vi "与副屏通信master.vi"() -> ()   [LabVIEW 2016, in "斯坦道多参数.lvlib"]
uses:
  <vilib>/NI/Modbus Library/API/Wrapper/Create TCP Master.vi
  <vilib>/NI/Modbus Library/API/master/Modbus Master.lvclass
  <vilib>/NI/Modbus Library/API/Wrapper/API Main.lvlib
  <vilib>/ptbypt/NI_PtbyPt.lvlib
panel:
  out "副屏启动命令":u16
  in  "停止 2":bool
  out "read values 2":u16[](array[numeric])
  in  "registers to write 2":u16[](array[numeric])
  out "error out 2":errorcluster caption="error out"
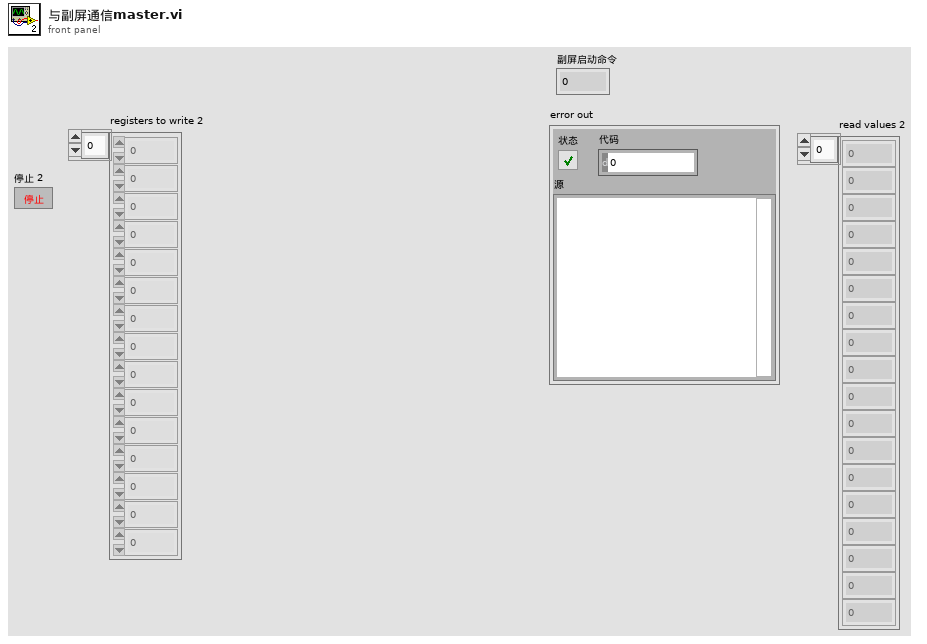
[diagram p1: front panel]
types:
  T1 = enum32{"Bad", "Idle", "Run top level", "Running"}
  T2 = cluster{"Boolean array[0]":bool, "Boolean array[1]":bool, "Boolean array[2]":bool, "Boolean array[3]":bool, "Boolean array[4]":bool, "Boolean array[5]":bool, "Boolean array[6]":bool, "Boolean array[7]":bool}
  T3 = cluster{"数据保存间隔":dbl, "保存组数":dbl, "水温标样值":dbl, "pH标样值":dbl, "溶解氧标样值":dbl, "电导率标样值":dbl, "浊度标样值":dbl, "pH启用":bool, "溶解氧启用":bool, "电导率启用":bool, "浊度启用":bool}
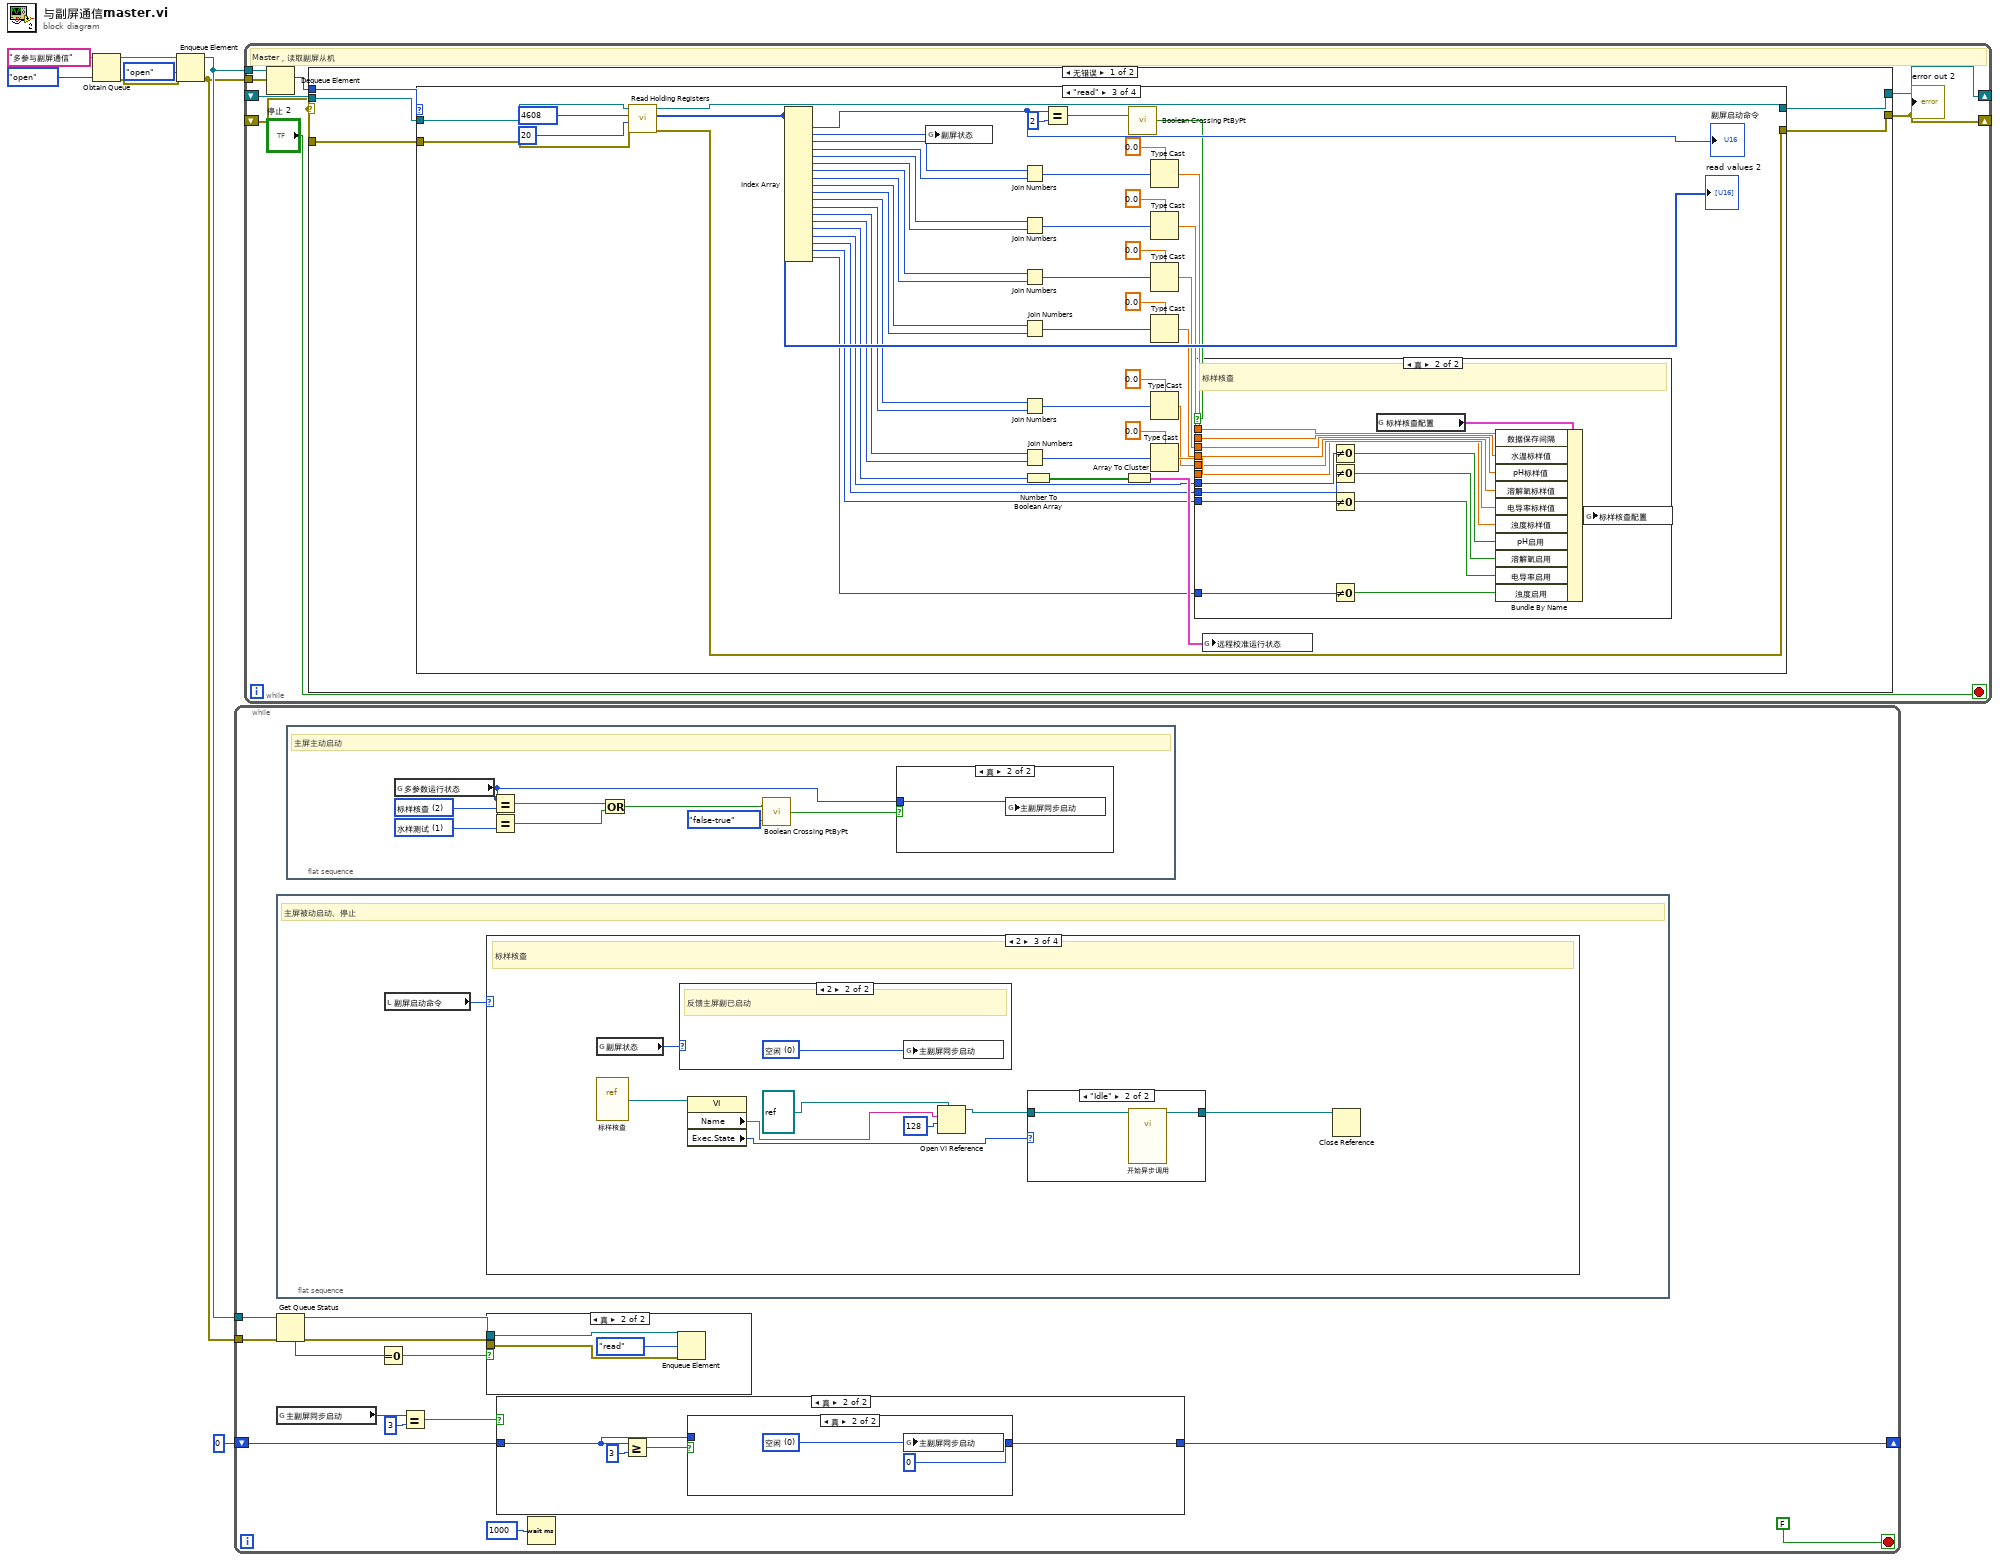
[diagram p0: block diagram]
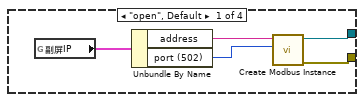
[diagram p2: hidden frame]
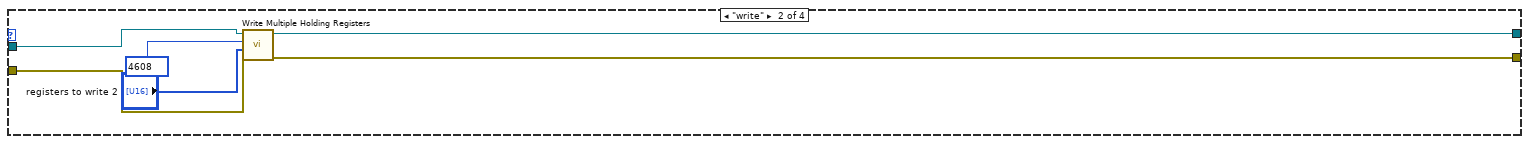
[diagram p3: hidden frame]
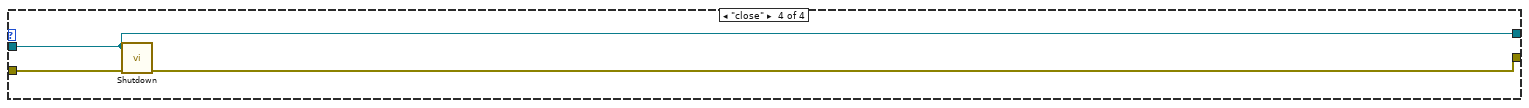
[diagram p5: hidden frame]
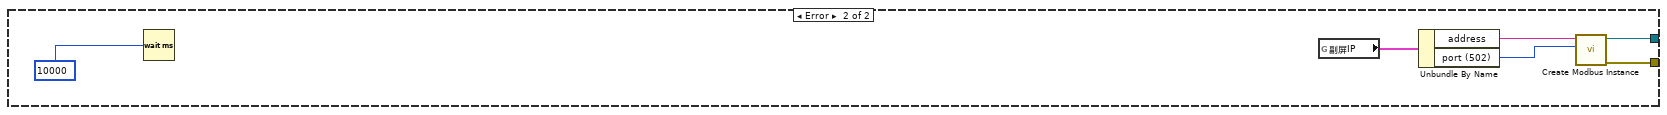
[diagram p6: hidden frame]
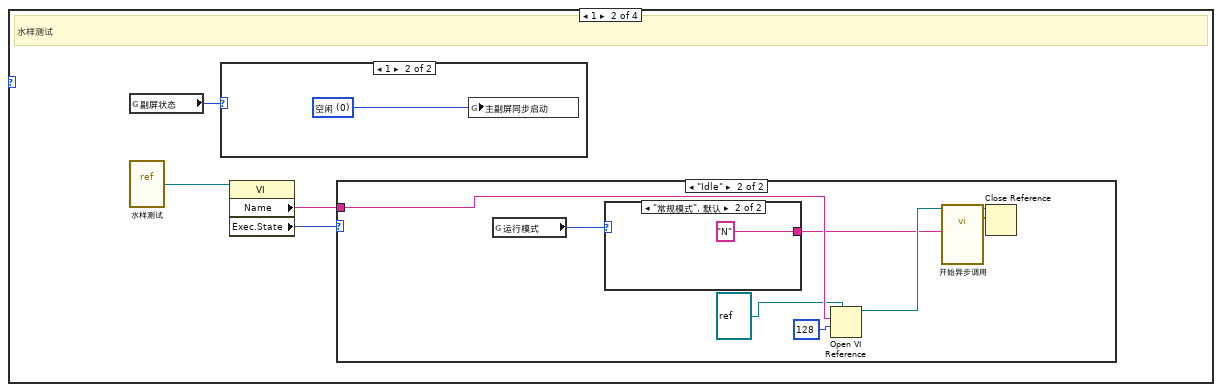
[diagram p8: hidden frame]
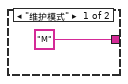
[diagram p11: hidden frame]
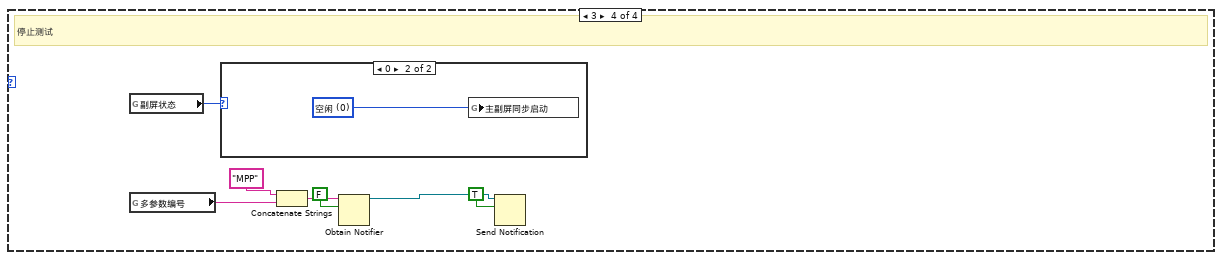
[diagram p14: hidden frame]
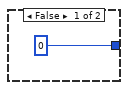
[diagram p16: hidden frame]
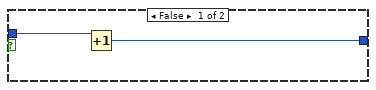
[diagram p17: hidden frame]
diagram:
  n1 = Obtain Queue(name (unnamed)="多参与副屏通信" ("名称（未命名）"), element data type=enum16{"open", "write", "read", "close"}."open") -> (queue out=w5:refnum<queue>, error out=w6:errorcluster)  [unwired: 3 in, 1 out]
  n2 = Enqueue Element(queue=w5, element=enum16{"open", "write", "read", "close"}."open", error in (no error)=w6) -> (queue out=w3:refnum<queue>, error out=w2:errorcluster)  [unwired: 1 in, 1 out]
  n3 = while {
    tunnel: w3 -> [w15]
    tunnel: w2 -> [w14]
    shift-right: [w9] -> _
    shift-left: u32 0 ("等待时间（毫秒）") -> [w10]
    stop <- FALSE stop-if-true
    n4 = flat-sequence {
      frame #0 {
        # "主屏被动启动、停止"
        n5 = local read "副屏启动命令"() -> (w22:u16)
        n6 = case shown="2" w22 {
          frame 0, Default {
          }
          frame 1 {
            # "水样测试"
            n7 = global read "多参数全局变量.vi" "副屏状态"() -> (w23:u16)
            n8 = vi-ref "水样测试.vi"() -> (w26:refnum<vi>)
            n9 = case shown="1" w23 {
              frame 0, Default {
              }
              frame 1 {
                w27 = u16 0 items=["空闲", "水样测试", "标样核查", "停止"] ("主副屏同步启动")
                n10 = global write "多参数全局变量.vi" "主副屏同步启动"(w27) -> ()
              }
            }
            n11 = property class="VI"(reference=w26) -> ("Name"=w24:string, "Exec.State"=w25:T1)  [unwired: 1 in, 2 out]
            n12 = case shown="\"Idle\"" w25 {
              tunnel: w24 -> [_ w32]
              frame "Bad", Default {
              }
              frame "Idle" {
                n13 = global read "多参数全局变量.vi" "运行模式"() -> (w30:enum16{"维护模式", "常规模式", "应急模式", "质控模式"})
                n14 = case shown="\"常规模式\", 默认" w30 {
                  tunnel: ["M" ("数据标记表") "N" ("数据标记表")] -> w29
                  frame "维护模式" {
                  }
                  frame "常规模式", Default {
                  }
                }
                n15 = Open VI Reference(type specifier VI Refnum (for type only)=refnum<vi> refnum, vi path=w32, options=128 ("选项")) -> (vi reference=w33:refnum<vi>)  [unwired: 3 in, 1 out]
                n16 = call-by-ref "开始异步调用"(reference=w33, "数据标记表"=w29) -> (reference out=w34:refnum<vi>, error out=w35:errorcluster)  [unwired: 12 in]
                n17 = Close Reference(reference=w34, error in (no error)=w35) -> ()  [unwired: 1 out]
              }
            }
          }
          frame 2 {
            # "标样核查"
            n18 = global read "多参数全局变量.vi" "副屏状态"() -> (w45:u16)
            n19 = vi-ref "标样核查.vi"() -> (w44:refnum<vi>)
            n20 = case shown="2" w45 {
              frame 0, Default {
              }
              frame 2 {
                w46 = u16 0 items=["空闲", "水样测试", "标样核查", "停止"] ("主副屏同步启动")
                # "反馈主屏副已启动"
                n21 = global write "多参数全局变量.vi" "主副屏同步启动"(w46) -> ()
              }
            }
            n22 = property class="VI"(reference=w44) -> ("Name"=w40:string, "Exec.State"=w42:T1)  [unwired: 1 in, 2 out]
            n23 = Open VI Reference(type specifier VI Refnum (for type only)=refnum<vi> refnum, vi path=w40, options=128 ("选项")) -> (vi reference=w39:refnum<vi>)  [unwired: 3 in, 1 out]
            n24 = case shown="\"Idle\"" w42 {
              tunnel: [w47 w49] -> w43
              tunnel: w39 -> [w47 w48]
              frame "Bad", Default {
              }
              frame "Idle" {
                n25 = call-by-ref "开始异步调用"(reference=w48) -> (reference out=w49:refnum<vi>)  [unwired: 13 in, 1 out]
              }
            }
            n26 = Close Reference(reference=w43) -> ()  [unwired: 1 in, 1 out]
          }
          frame 3 {
            # "停止测试"
            n27 = global read "多参数全局变量.vi" "副屏状态"() -> (w50:u16)
            n28 = global read "多参数全局变量.vi" "多参数编号"() -> (w53:string)
            n29 = case shown="0" w50 {
              frame 1, Default {
              }
              frame 0 {
                w57 = u16 0 items=["空闲", "水样测试", "标样核查", "停止"] ("主副屏同步启动")
                n30 = global write "多参数全局变量.vi" "主副屏同步启动"(w57) -> ()
              }
            }
            n31 = Concatenate Strings("MPP" ("名称（未命名）"), w53) -> (w54:string)
            n32 = Obtain Notifier(name (unnamed)=w54, notification data type=FALSE) -> (notifier out=w51:refnum<notifier>)  [unwired: 2 in, 2 out]
            n33 = Send Notification(notification=TRUE ("通知"), notifier=w51) -> ()  [unwired: 1 in, 2 out]
          }
        }
      }
    }
    n34 = Get Queue Status(queue=w15, error in (no error)=w14) -> (queue out=w17:refnum<queue>, error out=w18:errorcluster, # elements in queue=w16:i32)  [unwired: 1 in, 5 out]
    n35 = global read "多参数全局变量.vi" "主副屏同步启动"() -> (w13:u16)
    n36 = flat-sequence {
      frame #0 {
        w69 = u16 2 items=["空闲", "水样测试", "标样核查"] ("多参数运行状态")
        w72 = u16 1 items=["空闲", "水样测试", "标样核查"] ("多参数运行状态")
        # "主屏主动启动"
        n37 = global read "多参数全局变量.vi" "多参数运行状态"() -> (w68:u16)
        n38 = Equal?(x=w68, y=w69) -> (x = y?=w67:bool)
        n39 = Equal?(x=w68, y=w72) -> (x = y?=w73:bool)
        n40 = Or(x=w67, y=w73) -> (x .or. y?=w70:bool)
        n41 = call <vilib>:"Boolean Crossing PtByPt.vi"("direction"=enum16{"either", "false-true", "true-false"}."false-true", "input"=w70) -> ("crossing"=w71:bool)  [unwired: 1 in]
        n42 = case shown="真" w71 {
          tunnel: w68 -> [_ w75]
          frame False {
          }
          frame True {
            n43 = global write "多参数全局变量.vi" "主副屏同步启动"(w75) -> ()
          }
        }
      }
    }
    n44 = Equal To 0?(x=w16) -> (x = 0?=w19:bool)
    n45 = Equal?(x=w13, y=u16 3) -> (x = y?=w11:bool)
    n46 = case shown="真" w19 {
      tunnel: w17 -> [_ w77]
      tunnel: w18 -> [_ w76]
      frame False {
      }
      frame True {
        n47 = Enqueue Element(queue=w77, element=enum16{"open", "write", "read", "close"}."read", error in (no error)=w76) -> ()  [unwired: 1 in, 3 out]
      }
    }
    n48 = case shown="真" w11 {
      tunnel: w10 -> [_ w61]
      tunnel: [u32 0 w62] -> w9
      frame False {
      }
      frame True {
        n49 = Greater Or Equal?(x=w61, y=u32 3) -> (x >= y?=w59:bool)
        n50 = case shown="真" w59 {
          tunnel: [w64 u32 0] -> w62
          tunnel: w61 -> [w63 _]
          frame False {
            n51 = Increment(x=w63) -> (x+1=w64:u32)
          }
          frame True {
            w66 = u16 0 items=["空闲", "水样测试", "标样核查", "停止"] ("主副屏同步启动")
            n52 = global write "多参数全局变量.vi" "主副屏同步启动"(w66) -> ()
          }
        }
      }
    }
    n53 = Wait (ms)(milliseconds to wait=u32 1000 ("等待时间（毫秒）")) -> ()  [unwired: 1 out]
  }
  n54 = while {
    shift-right: [w83] -> _
    shift-left: _ -> [w85]
    shift-right: [w84] -> _
    shift-left: _ -> [w82]
    tunnel: w3 -> [w81]
    tunnel: w2 -> [w80]
    stop <- "停止 2" stop-if-true
    # "Master，读取副屏从机"
    n55 = Dequeue Element(queue=w81, error in (no error)=w80) -> (element=w79:enum16{"open", "write", "read", "close"})  [unwired: 1 in, 3 out]
    n56 = case shown="无错误" w82 {
      tunnel: w85 -> [w91 _]
      tunnel: w82 -> [w90 _]
      tunnel: [w89 w175] -> w84
      tunnel: [w88 w176] -> w83
      tunnel: w79 -> [w87 _]
      frame No Error {
        n57 = case shown="\"read\"" w87 {
          tunnel: w91 -> [_ w102 w113 w170]
          tunnel: w90 -> [_ w100 w112 w169]
          tunnel: [w95 w97 w110 w168] -> w89
          tunnel: [w96 w98 w111 w170] -> w88
          frame "open", Default {
            n58 = global read "多参数全局变量.vi" "副屏IP"() -> (w94:cluster{"address":string, "port (502)":u16})
            n59 = Unbundle By Name(w94) -> ("address"=w93:string, "port (502)"=w92:u16)
            n60 = call-poly <vilib>:"Create Modbus Instance.vi"("port (502)"=w92, "address"=w93) -> ("error out"=w95:errorcluster, "TCP master instance"=w96:refnum<class "Modbus Master.lvclass">)  [unwired: 8 in]
          }
          frame "write" {
            n61 = call-dynamic "Write Multiple Holding Registers.vi"("error in"=w100, "registers to write"="registers to write 2", "starting address"=u16 4608 ("write starting address"), "Modbus master in"=w102) -> ("error out"=w97:errorcluster, "Modbus master out"=w98:refnum<class "Modbus Master.lvclass">)  [unwired: 6 in]
          }
          frame "read" {
            n62 = call-dynamic "Read Holding Registers.vi"("error in"=w112, "number of inputs"=u16 20 ("read count"), "starting address"=u16 4608 ("write starting address"), "Modbus master in"=w113) -> ("error out"=w110:errorcluster, "register values"=w149:u16[], "Modbus master out"=w111:refnum<class "Modbus Master.lvclass">)  [unwired: 5 in]
            "read values 2" <- w149
            n63 = Index Array(array=w149) -> (element #1=w150:u16, element #2=w151:u16, element #3=w118:u16, element #4=w119:u16, element #5=w125:u16, element #6=w124:u16, element #7=w129:u16, element #8=w128:u16, element #9=w134:u16, element #10=w135:u16, element #11=w142:u16, element #12=w143:u16, element #13=w144:u16, element #14=w145:u16, element #15=w107:u16, element #16=w106:u16, element #17=w105:u16, element #18=w104:u16, element #19=w103:u16)  [unwired: 19 in]
            "副屏启动命令" <- w150
            n64 = global write "多参数全局变量.vi" "副屏状态"(w151) -> ()
            n65 = Join Numbers(hi=w118, lo=w119) -> ((hi.lo)=w117:u32)
            n66 = Join Numbers(hi=w125, lo=w124) -> ((hi.lo)=w122:u32)
            n67 = Join Numbers(hi=w129, lo=w128) -> ((hi.lo)=w127:u32)
            n68 = Join Numbers(hi=w134, lo=w135) -> ((hi.lo)=w132:u32)
            n69 = Join Numbers(hi=w142, lo=w143) -> ((hi.lo)=w137:u32)
            n70 = Join Numbers(hi=w144, lo=w145) -> ((hi.lo)=w139:u32)
            n71 = Number To Boolean Array(number=w107) -> (Boolean array=w109:bool[])
            n72 = Equal?(x=w150, y=u16 2) -> (x = y?=w147:bool)
            n73 = Array To Cluster(array=w109) -> (cluster=w108:T2)
            n74 = call <vilib>:"Boolean Crossing PtByPt.vi"("input"=w147) -> ("crossing"=w148:bool)  [unwired: 2 in]
            n75 = Type Cast(type=sgl 0.0, x=w117) -> (*(type *) &x=w120:sgl)
            n76 = Type Cast(type=sgl 0.0, x=w122) -> (*(type *) &x=w123:sgl)
            n77 = Type Cast(type=sgl 0.0, x=w127) -> (*(type *) &x=w130:sgl)
            n78 = Type Cast(type=sgl 0.0, x=w132) -> (*(type *) &x=w133:sgl)
            n79 = Type Cast(type=sgl 0.0, x=w137) -> (*(type *) &x=w140:sgl)
            n80 = Type Cast(type=sgl 0.0, x=w139) -> (*(type *) &x=w141:sgl)
            n81 = case shown="真" w148 {
              tunnel: w120 -> [_ w165]
              tunnel: w123 -> [_ w164]
              tunnel: w130 -> [_ w163]
              tunnel: w133 -> [_ w162]
              tunnel: w140 -> [_ w161]
              tunnel: w141 -> [_ w160]
              tunnel: w106 -> [_ w159]
              tunnel: w105 -> [_ w155]
              tunnel: w104 -> [_ w157]
              tunnel: w103 -> [_ w156]
              frame False {
              }
              frame True {
                # "标样核查"
                n82 = Not Equal To 0?(x=w159) -> (x != 0?=w158:bool)
                n83 = Not Equal To 0?(x=w155) -> (x != 0?=w154:bool)
                n84 = Not Equal To 0?(x=w157) -> (x != 0?=w153:bool)
                n85 = Not Equal To 0?(x=w156) -> (x != 0?=w152:bool)
                n86 = global read "断电保存变量.vi" "标样核查配置"() -> (w167:T3)
                n87 = Bundle By Name(cluster=w167, "数据保存间隔"=w165, "水温标样值"=w164, "pH标样值"=w163, "溶解氧标样值"=w162, "电导率标样值"=w161, "浊度标样值"=w160, "pH启用"=w158, "溶解氧启用"=w154, "电导率启用"=w153, "浊度启用"=w152) -> (w166:T3)
                n88 = global write "断电保存变量.vi" "标样核查配置"(w166) -> ()
              }
            }
            n89 = global write "多参数全局变量.vi" "远程校准运行状态"(w108) -> ()
          }
          frame "close" {
            n90 = call-dynamic "Shutdown.vi"("error in"=w169, "Modbus master in"=w170) -> ("error out"=w168:errorcluster)  [unwired: 9 in]
          }
        }
      }
      frame Error {
        n91 = Wait (ms)(milliseconds to wait=u32 10000 ("等待时间（毫秒）")) -> ()  [unwired: 1 out]
        n92 = global read "多参数全局变量.vi" "副屏IP"() -> (w173:cluster{"address":string, "port (502)":u16})
        n93 = Unbundle By Name(w173) -> ("address"=w172:string, "port (502)"=w171:u16)
        n94 = call-poly <vilib>:"Create Modbus Instance.vi"("port (502)"=w171, "address"=w172) -> ("error out"=w175:errorcluster, "TCP master instance"=w176:refnum<class "Modbus Master.lvclass">)  [unwired: 8 in]
      }
    }
    "error out 2" <- w84
  }
